vi "AnOperation.vi"(8 "error in (no error)":errorcluster, 11 "Creator":refnum<class "Creator.lvclass">) -> (0 "error out":errorcluster, 2 "ResultString":string, 3 "Creator":refnum<class "Creator.lvclass">)   [LabVIEW 2020, in "FactoryMethod.lvlib" / "FactoryMethodLazyEvaluation.lvlib" / "Creator.lvclass"]
uses:
  Creator.lvclass
  Product/Product.lvclass
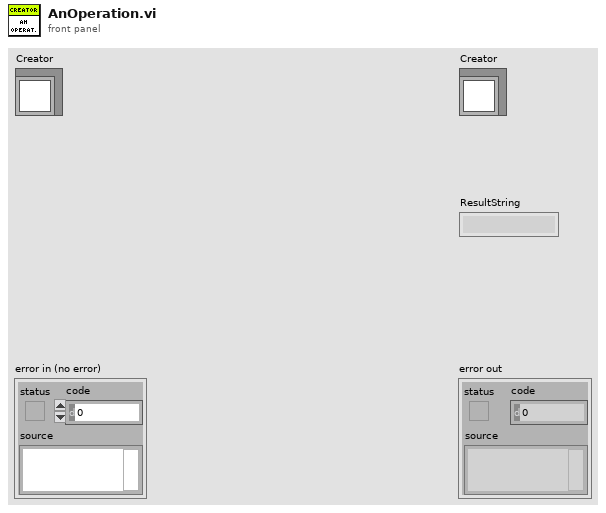
[diagram p1: front panel]
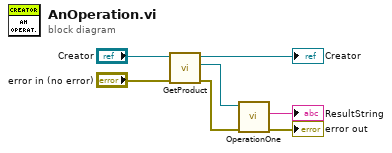
[diagram p0: block diagram]
diagram:
  n1 = call "GetProduct.vi"("error in"="error in (no error)", "Creator"="Creator") -> ("error out"=w4:errorcluster, "Product"=w3:refnum<class "Product.lvclass">, "Creator"=→"Creator":refnum<class "Creator.lvclass">)  [unwired: 7 in]
  n2 = call-dynamic "OperationOne.vi"("error in (no error)"=w4, "Product in"=w3) -> ("error out"=→"error out":errorcluster, "ResultString"=→"ResultString":string)  [unwired: 7 in, 1 out]
